vi "Set Angle.vi"(6 "Axis":T1, 8 "error in (no error)":errorcluster, 9 "Rate (°)/min)":dbl, 10 "Angle (°)":dbl, 11 "instrument.PPMS":refnum<class "instrument.PPMS.lvclass">) -> (0 "error out":errorcluster, 3 "instrument.PPMS out":refnum<class "instrument.PPMS.lvclass">)   [LabVIEW 2019, in "instrument.PPMS.lvclass"]
uses:
  instrument.PPMS.lvclass
  e647ebb3-b22b-49f8-a713-7ef316bda7c2.vi/247d8595-c488-48cb-b3dc-7351fa439d49.vi
  e647ebb3-b22b-49f8-a713-7ef316bda7c2.vi/e1100621-a18b-4c0b-b301-6ab00cbab1fb.vi
  e647ebb3-b22b-49f8-a713-7ef316bda7c2.vi/e1100621-a18b-4c0b-b301-6ab00cbab1fb.vi/ddc7ecc4-f6e6-4bb2-95e6-d490f4452c5c.vi
  e647ebb3-b22b-49f8-a713-7ef316bda7c2.vi/e1100621-a18b-4c0b-b301-6ab00cbab1fb.vi/950473b1-726b-41a3-a6af-9dd795e86957.vi
  <userlib>/LevyLab/Levylab Instruments/SMOs/RemoteControl/API/Remote Client.vi
  <vilib>/JDP Science/JSONtext/JSON text to Variant.vi
  <vilib>/JDP Science/JSONtext/LVClass Serializer/JSONtext LVClass Serializer.lvclass
  <userlib>/LevyLab/Levylab Instruments/Instrument Types/Cryostat/Typedefs/Rotator Axis--Enum.ctl
  <userlib>/LevyLab/Levylab Instruments/Instrument Types/Cryostat/Instrument.Cryostat.lvclass
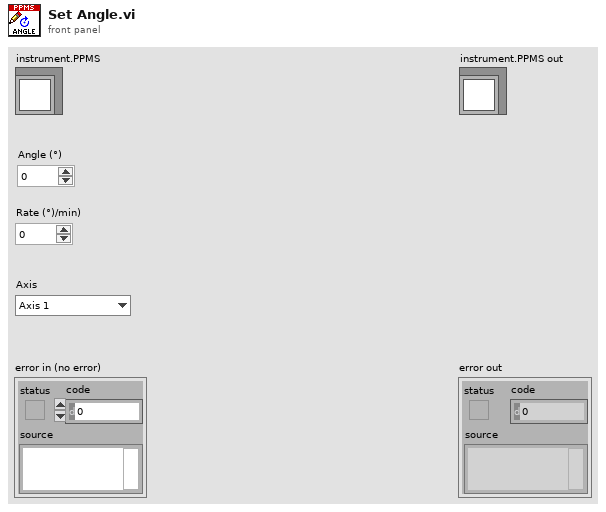
[diagram p1: front panel]
types:
  T1 = typedef "Instrument.Cryostat.lvclass/Rotator Axis--Enum.ctl" = enum16{"Axis 1", "Axis 2"}
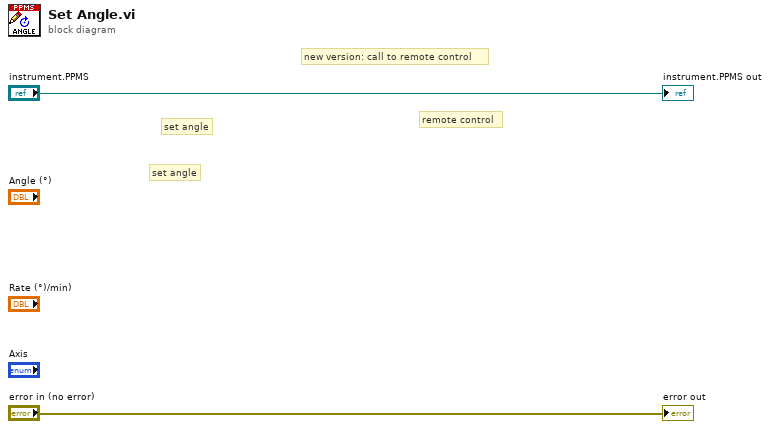
[diagram p0: block diagram]
diagram:
  # "remote control"
  # "set angle"
  # "set angle"
  # "new version: call to remote control"
  "error out" <- "error in (no error)"
  "instrument.PPMS out" <- "instrument.PPMS"
